vi "HandleTrigger.vi"(8 "error in (no error)":errorcluster, 9 "SyncBox transition":bool, 10 "SyncBox status":bool, 11 "Acquisition in":refnum<class "Acquisition.lvclass">) -> (0 "error out":errorcluster, 3 "Acquisition out":refnum<class "Acquisition.lvclass">)   [LabVIEW 2018, in "Acquisition.lvclass"]
uses:
  Acquisition.lvclass
  C:/Users/devstaff/sparc4/s4gui/Versao ZeroMQ REQ-REP/SPARC4_GUI -20241111/Server/Server.lvclass
  Server/Server.lvclass/Server.ctl
  Interface/Interface.lvclass/Interface.ctl
  Channel/Channel.lvclass
  Interface/Interface.lvclass
  StateMachine/State Machine.lvclass
  Server/Server.lvclass
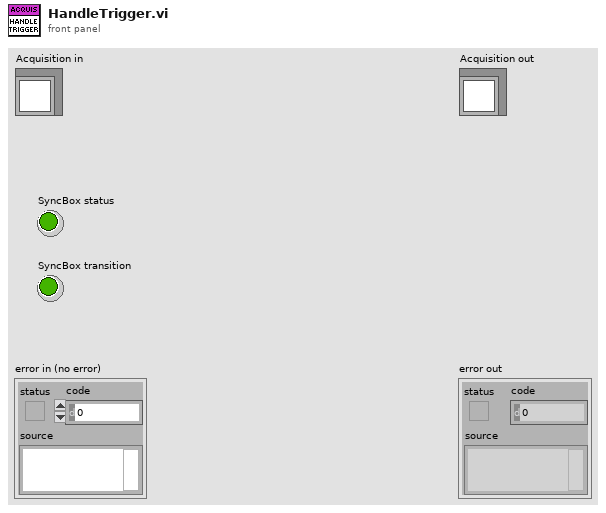
[diagram p1: front panel]
types:
  T1 = cluster{"ACQUISITION_MODE":u8, "TRIGGER_MODE":u8, "READ_MODE":u8, "PREAMP":u8, "READOUT_RATE":u8, "VERTICAL_SHIFT_SPEED":u8, "EM_MODE":u8, "EM_GAIN":u16, "SHUTTER_MODE":u8, "SHUTTER_TTL":u8, "SHUTTER_OPENING_TIME":u16, "SHUTTER_CLOSING_TIME":u16, "VBIN":u16, "HBIN":u16, "INITIAL_LINE":u16, "INITIAL_COLUMN":u16, "FINAL_LINE":u16, "FINAL_COLUMN":u16, "FRAME_TRANSFER":bool, "VERTICAL_CLOCK_VOLTAGE":u8, "AD_CHANNEL":u32}
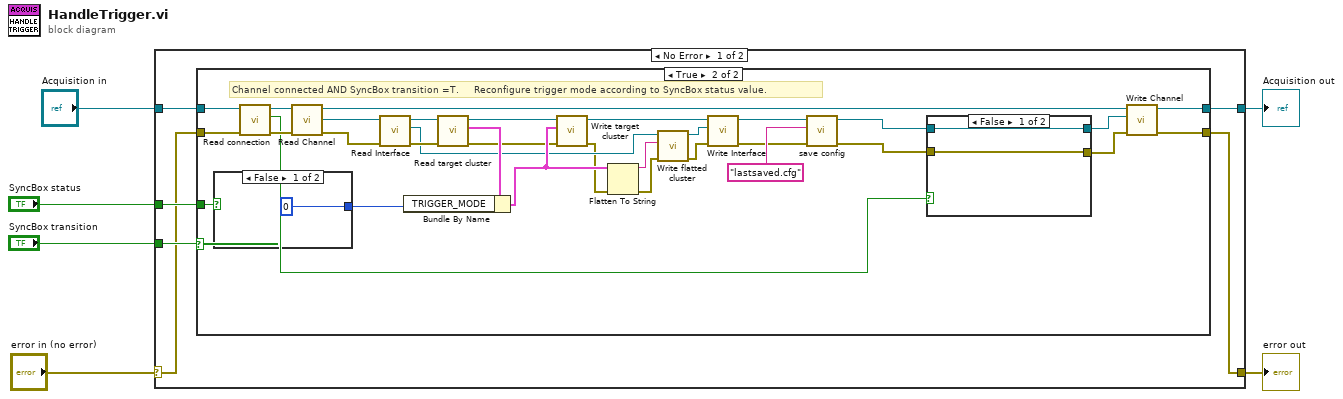
[diagram p0: block diagram]
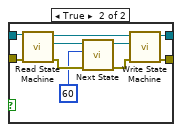
[diagram p3: hidden frame]
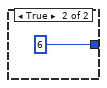
[diagram p4: hidden frame]
diagram:
  n1 = case shown="No Error" "error in (no error)" {
    selector: "error in (no error)" -> [w8 w62]
    tunnel: [w10 w62] -> w5
    tunnel: [w11 w61] -> w3
    tunnel: "Acquisition in" -> [w7 w61]
    tunnel: "SyncBox status" -> [w12 _]
    tunnel: "SyncBox transition" -> [w9 _]
    frame No Error {
      n2 = case shown="True" w9 {
        tunnel: w12 -> [_ w35]
        tunnel: w7 -> [w14 w28]
        tunnel: [w14 w36] -> w11
        tunnel: w8 -> [w13 w26]
        tunnel: [w13 w34] -> w10
        frame False {
          # "Channel disconnected OR SyncBox transition=F.     Nothing to do."
        }
        frame True {
          # "Channel connected AND SyncBox transition =T.     Reconfigure trigger mode according to SyncBox status value."
          n3 = case shown="False" w35 {
            tunnel: [u8 0 ("TRIGGER_MODE") u8 6 ("TRIGGER_MODE")] -> w37
            frame False {
            }
            frame True {
            }
          }
          n4 = call "Read connection.vi"("error in (no error)"=w26, "Server in"=w28) -> ("error out"=w25:errorcluster, "connection"=w24:bool, "Server out"=w27:refnum<class "Acquisition.lvclass">)  [unwired: 7 in]
          n5 = call-dynamic "Read Channel.vi"("error in (no error)"=w25, "Acquisition in"=w27) -> ("error out"=w42:errorcluster, "Channel.lvclass"=w41:refnum<class "Channel.lvclass">, "Acquisition out"=w29:refnum<class "Acquisition.lvclass">)  [unwired: 7 in]
          n6 = call-dynamic "Read Interface.vi"("error in (no error)"=w42, "Channel in"=w41) -> ("error out"=w22:errorcluster, "Interface.lvclass"=w18:refnum<class "Interface.lvclass">, "Channel out"=w23:refnum<class "Channel.lvclass">)  [unwired: 7 in]
          n7 = call-dynamic "Read target cluster.vi"("error in (no error)"=w22, "Channel in"=w23) -> ("error out"=w15:errorcluster, "target cluster"=w21:T1, "Channel out"=w19:refnum<class "Channel.lvclass">)  [unwired: 7 in]
          n8 = Bundle By Name(cluster=w21, "TRIGGER_MODE"=w37) -> (w20:T1)
          n9 = call-dynamic "Write target cluster.vi"("error in (no error)"=w15, "target cluster"=w20, "Channel in"=w19) -> ("error out"=w16:errorcluster, "Channel out"=w17:refnum<class "Channel.lvclass">)  [unwired: 7 in]
          n10 = Flatten To String(anything=w20, error in (no error)=w16) -> (data string=w46:string, error out=w45:errorcluster)  [unwired: 2 in, 1 out]
          n11 = call "Write flatted cluster.vi"("error in (no error)"=w45, "flatted cluster"=w46, "Interface in"=w18) -> ("error out"=w43:errorcluster, "Interface out"=w44:refnum<class "Interface.lvclass">)  [unwired: 7 in]
          n12 = call-dynamic "Write Interface.vi"("error in (no error)"=w43, "Interface.lvclass"=w44, "Channel in"=w17) -> ("error out"=w38:errorcluster, "Channel out"=w39:refnum<class "Channel.lvclass">)  [unwired: 7 in]
          n13 = call-dynamic "save config.vi"("error in (no error)"=w38, "file config"="lastsaved.cfg" ("cfg file name"), "Channel in"=w39) -> ("error out"=w31:errorcluster, "Channel out"=w33:refnum<class "Channel.lvclass">)  [unwired: 7 in]
          n14 = case shown="False" w24 {
            tunnel: w33 -> [w48 w55]
            tunnel: [w48 w53] -> w32
            tunnel: w31 -> [w47 w52]
            tunnel: [w47 w51] -> w30
            frame False {
            }
            frame True {
              n15 = call-dynamic "Read State Machine.vi"("error in (no error)"=w52, "Device in"=w55) -> ("error out"=w58:errorcluster, "State Machine.lvclass"=w50:refnum<class "State Machine.lvclass">, "Device out"=w54:refnum<class "Channel.lvclass">)  [unwired: 7 in]
              n16 = call "Next State.vi"("error in (no error)"=w58, "New_State"=60, "State Machine in"=w50) -> ("error out"=w57:errorcluster, "State Machine out"=w49:refnum<class "State Machine.lvclass">)  [unwired: 7 in]
              n17 = call-dynamic "Write State Machine.vi"("error in (no error)"=w57, "State Machine.lvclass"=w49, "Device in"=w54) -> ("error out"=w51:errorcluster, "Device out"=w53:refnum<class "Channel.lvclass">)  [unwired: 7 in]
            }
          }
          n18 = call-dynamic "Write Channel.vi"("error in (no error)"=w30, "Channel.lvclass"=w32, "Acquisition in"=w29) -> ("error out"=w34:errorcluster, "Acquisition out"=w36:refnum<class "Acquisition.lvclass">)  [unwired: 7 in]
        }
      }
    }
    frame Error {
    }
  }
  "error out" <- w5
  "Acquisition out" <- w3
